vi "Autonomous Independent.vi"() -> ()   [LabVIEW 2023]
doc: "This VI is called when autonomous begins, and will automatically be terminated when autonomous ends. You can carry out timed or sensor driven robot movement independently without needing to return to the caller."
uses:
  ctrl defs/ctrl robot swerve dims.ctl
  ctrl defs/ctrl AUTO SIMPLE STEP.ctl
  <vilib>/Rock Robotics/WPI/Utilities/WPI_GetSetVariantRefNum.vi
  <vilib>/Rock Robotics/Network Tables/NT Read String.vi
  <vilib>/Rock Robotics/Network Tables/NT Write Numeric Array.vi
  Global odometry.vi
  Global INIT.vi
  <vilib>/Rock Robotics/WPI/ThirdParty/JAS_Junk/TrajLib/Trajectory_Library.lvlib
  <vilib>/Rock Robotics/Network Tables/NT Write Boolean.vi
panel:
  in  "Tab Control":T1(tab)
  in  "leg 1 distance (ft)":dbl=1.06 format="%#_13g"
  in  "leg 1\nVBus":dbl=0.5 format="%#_13g"
  in  "leg 2 distance (ft)":dbl=8.0 format="%#_13g"
  in  "leg 2\nVBus":dbl=0.5 format="%#_13g"
  in  "DRIVE BRNG (deg)":dbl=60.0 min=0.0 max=90.0 format="%#_13g"
  in  "DRIVE CTR-STAGE (ft)":dbl=15.0 caption="distance wall to center stage (in feet)" min=0.02 max=27.0 step=0.02 format="%.2f"
  in  "DRIVE CTR-STAGE %VBus":dbl=0.5499999999999999 caption="drive center-stage throttle %" min=0.02 max=0.7 step=0.01 format="%.2f"
  in  "DRIVE MID-CT (ft)":dbl=25.76 caption="distance wall to mid-court (in feet)" min=0.02 max=27.0 step=0.02 format="%.2f"
  in  "DRIVE MID-CT %VBus":dbl=0.65 caption="drive mid-court throttle %" min=0.02 max=0.7 step=0.01 format="%.2f"
  in  "DRIVE OUT %VBus":dbl=0.5 caption="drive away throttle %" min=0.02 max=0.7 step=0.01 format="%.2f"
  in  "DRIVE OUT (ft)":dbl=8.0 caption="SPEAKER front to NOTE (in feet)" min=0.02 max=25.0 step=0.02 format="%.2f"
  in  "delay to wait to\nSHOOT (ms)":u32=1500
  in  "pause after\ndrive out (ms)":u32=500
  in  "DRIVE IN (ft)":dbl=8.0 caption="distance to return to SPEAKER (in feet)" min=0.02 max=25.0 step=0.02 format="%.2f"
  in  "DRIVE IN %VBus":dbl=0.4 caption="drive return throttle %" min=0.02 max=0.7 step=0.01 format="%.2f"
  out "ROBOT frame dims":T2={"width"=30.0, "depth"=30.0}
  in  "bumper thickness (in)":dbl=3.25 format="%#_13g"
  out "POS after (rev)":dbl[](array[numeric])
  out "POS start (rev)":dbl[](array[numeric])
  out "distance\ntravel (in)":dbl[](array[numeric])
  out "revs moved":dbl[](array[numeric])
  out "inches\nper rev":dbl
  out "YRPHfH start":T3={"Yaw"=129.52, "Roll"=0.02, "Pitch"=-0.05, "Heading"=270.74, "Fused Heading"=129.25}
  out "YRPHfH after first leg":T3={"Yaw"=129.52, "Roll"=0.02, "Pitch"=-0.05, "Heading"=270.74, "Fused Heading"=129.25}
  out "YRPHfH end":T3={"Yaw"=129.52, "Roll"=0.02, "Pitch"=-0.05, "Heading"=270.74, "Fused Heading"=129.25}
  out "overall change":T3
  out "change from leg 1 to 2":T3
  out "Milliseconds":u16
  out "av vel (in/s)":dbl[](array[numeric])
  # "ANGLED PROGRAMS from SUB-WOOFER sides"
  # "DISTANCES:\n\nGO-LINE:\n    6.34 ft from driver's wall\n    3.33 ft from sub-woofer\n\nNOTE line:\n    9.67 ft from driver's wall\n    6.65 ft from sub-woofer\n\nCENTER-STAGE line:\n    19.27 ft from driver's wall\n\nMID-COURT:\n     27.22 ft from driver's wall\n\nROBOT is 30 x 30 with 3.5\" bumpers\n37 x 37 overall; 18.5\" to center"
  # "Be sure to right-click and choose Data Operations>>Make Current Value default if you want to save the array values with the VI"
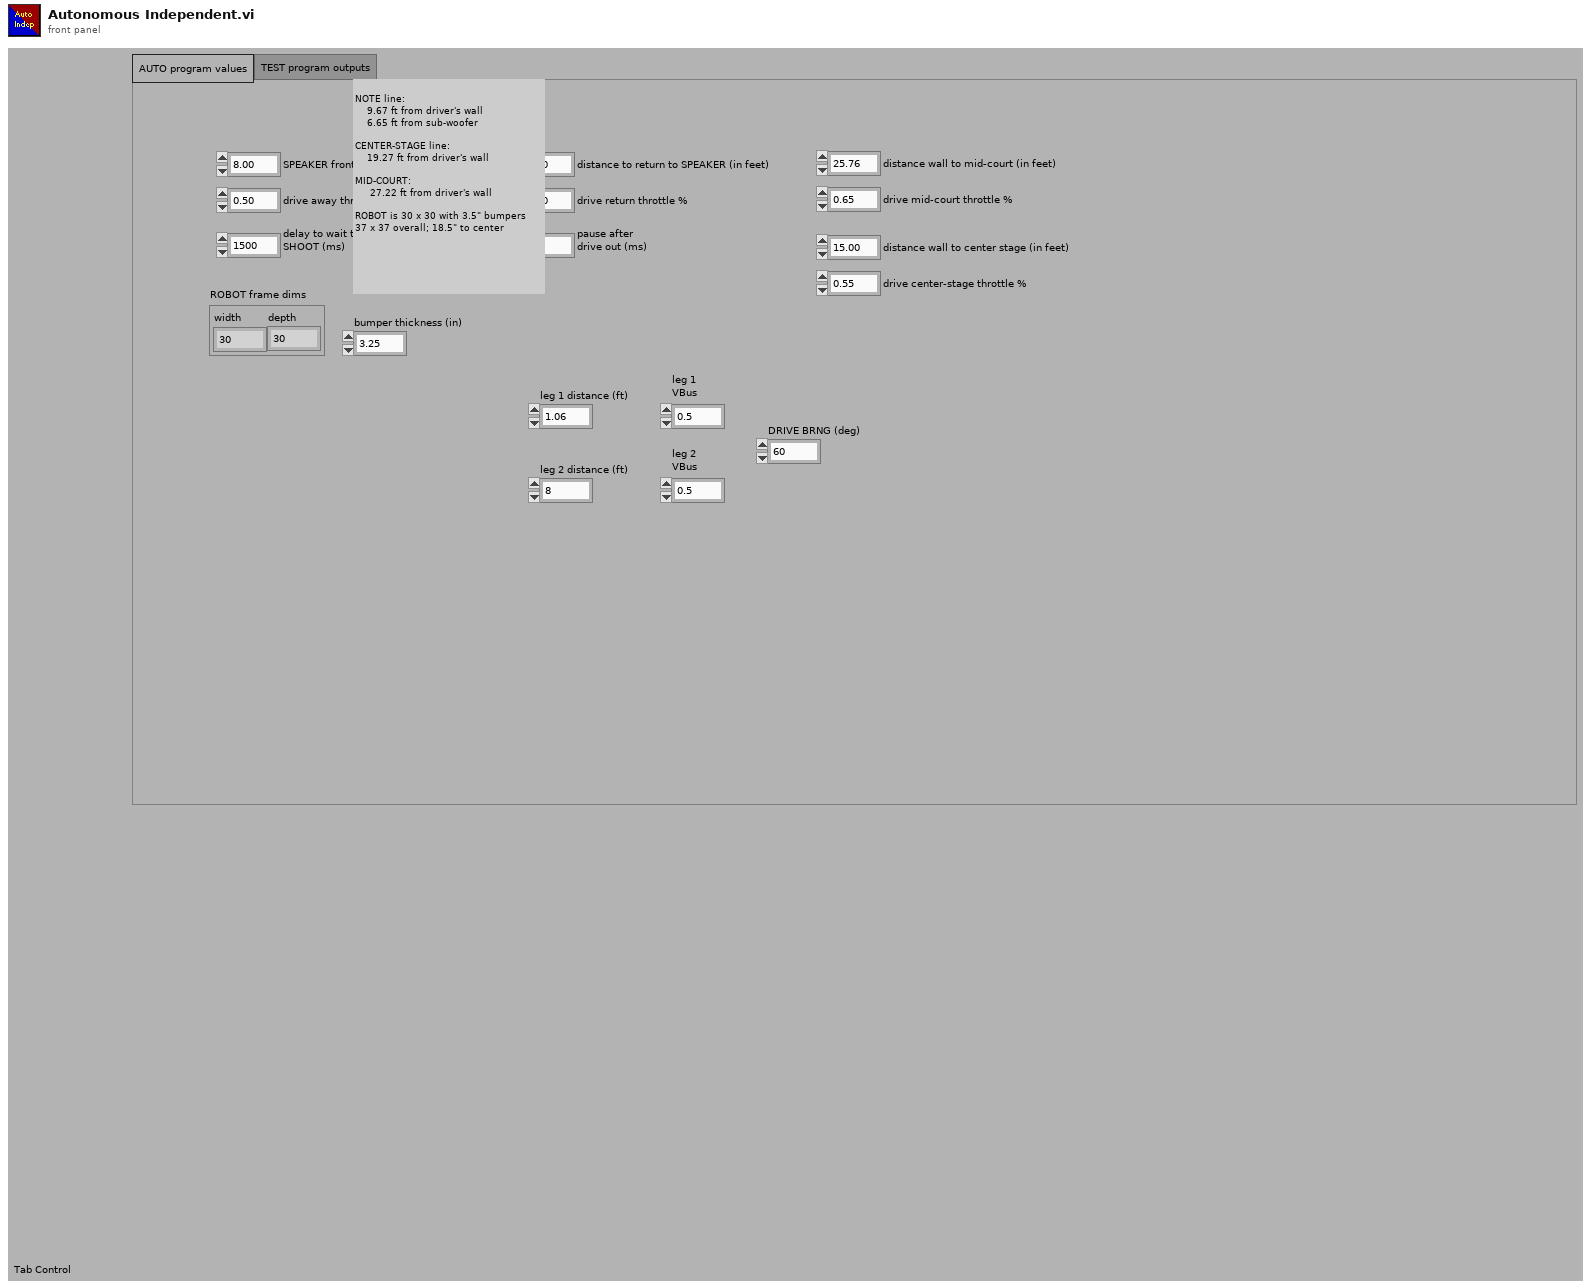
[diagram p1: front panel]
types:
  T1 = enum32{"AUTO program values", "TEST program outputs"}
  T2 = typedef "ctrl robot swerve dims.ctl" = cluster{"width":dbl, "depth":dbl}
  T3 = cluster{"Yaw":dbl, "Roll":dbl, "Pitch":dbl, "Heading":dbl, "Fused Heading":dbl}
  T4 = typedef "WPI_JoystickDevRef.ctl" = cluster{"Device":T5}
  T5 = typedef "WPI_JoystickDeviceEnum.ctl" = enum16{"USB 0", "USB 1", "USB 2", "USB 3", "USB 4", "USB 5"}
  T6 = typedef "ctrl AUTO SIMPLE STEP.ctl" = cluster{"SHOOT\nFIRST":bool, "wait to\nSHOOT (ms)":u32, "run\nINTAKE":bool, "DRIVE BRNG (deg)":dbl, "DRIVE OUT\nVBus":dbl, "TIME to\nDRIVE OUT (ms)":u32, "pause after\ndrive out (ms)":u32, "SHOOT\nAGAIN":bool, "DRIVE IN\nVBus":dbl, "TIME to\nDRIVE IN (ms)":u32}
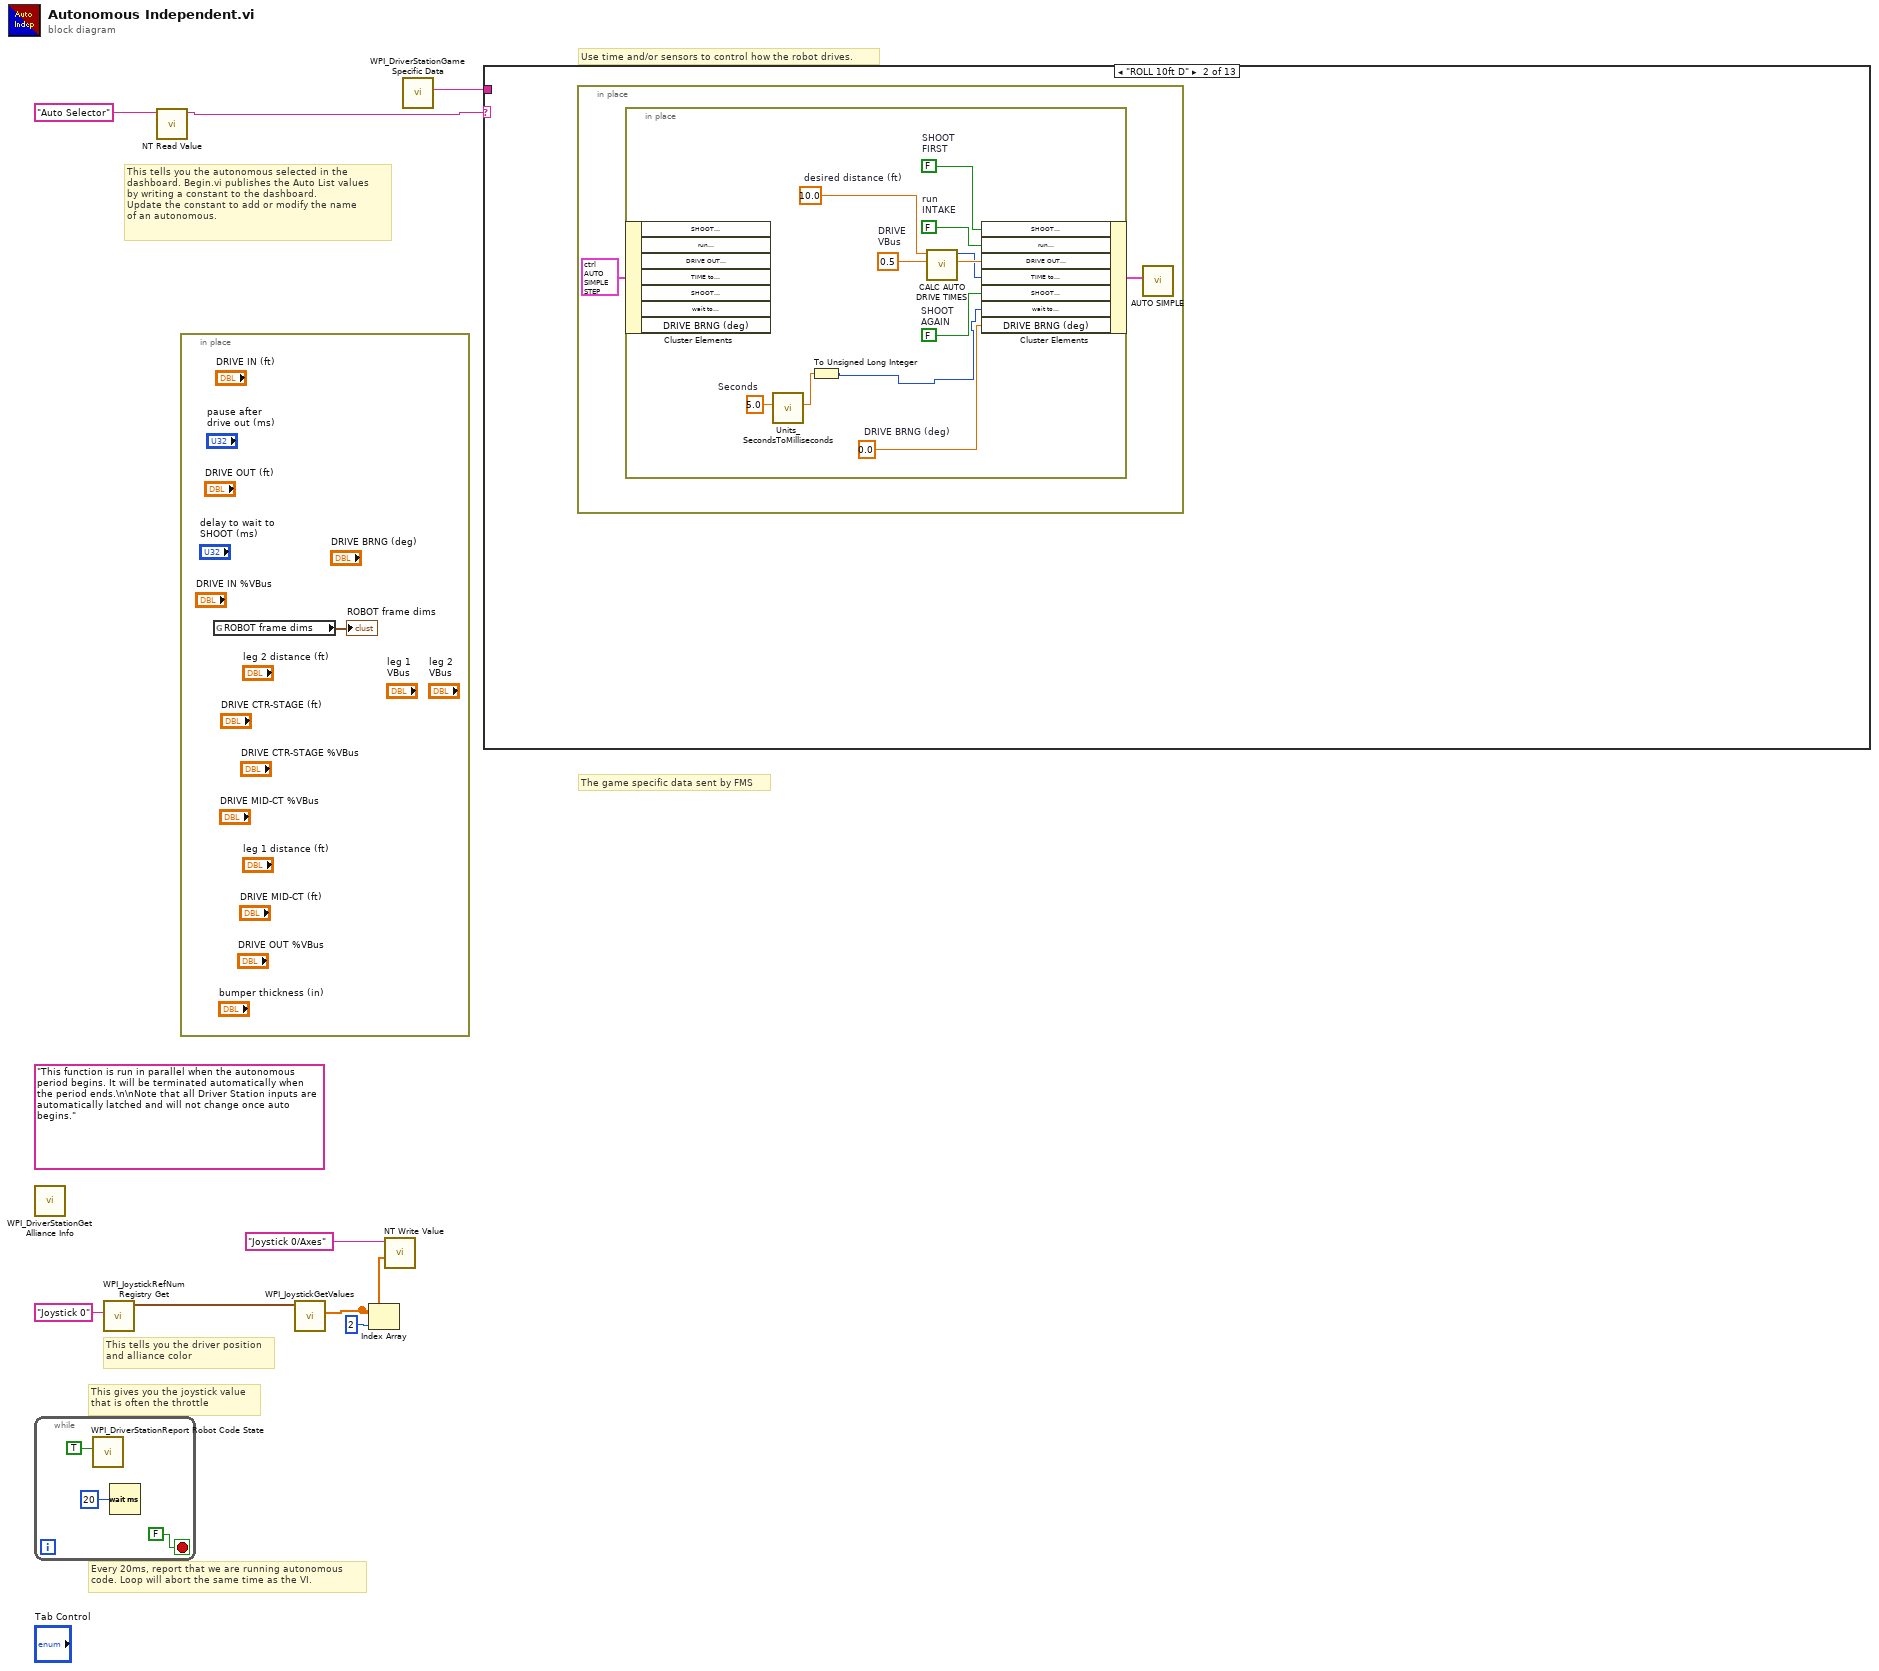
[diagram p0: block diagram]
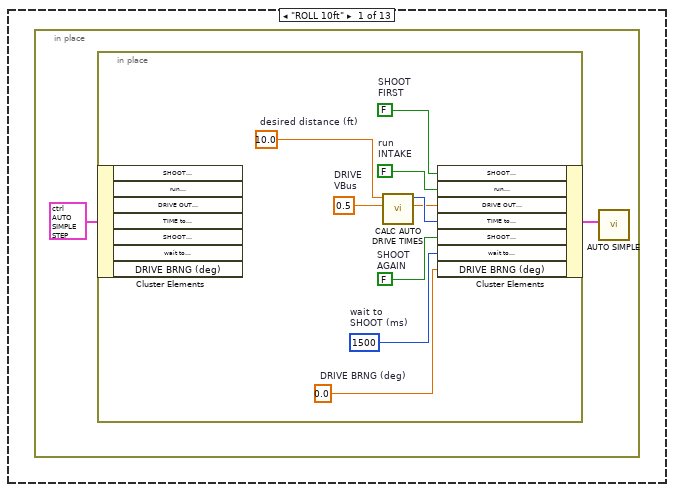
[diagram p2: hidden frame]
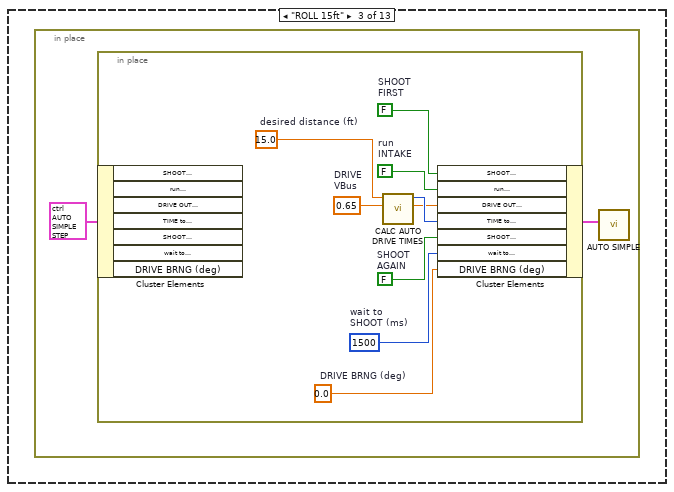
[diagram p3: hidden frame]
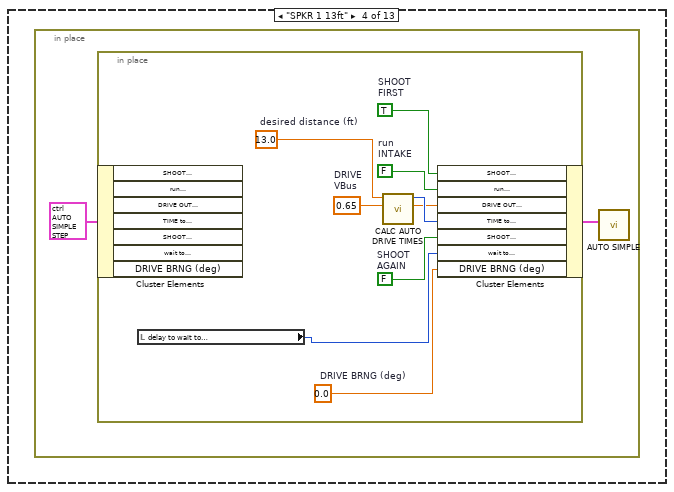
[diagram p4: hidden frame]
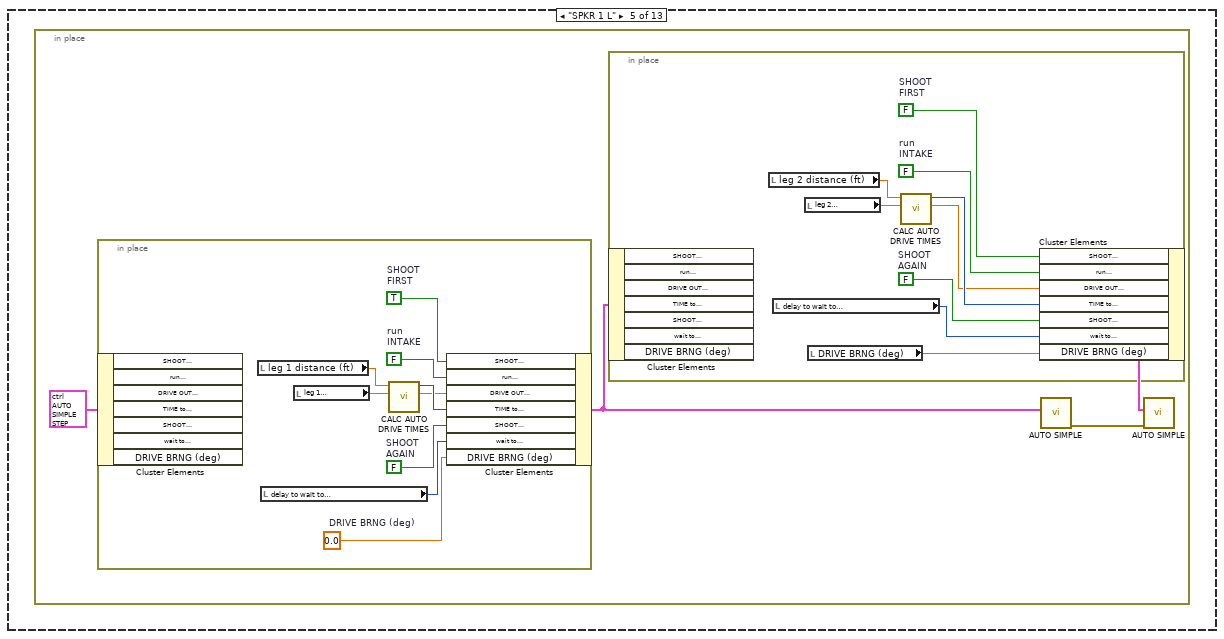
[diagram p5: hidden frame]
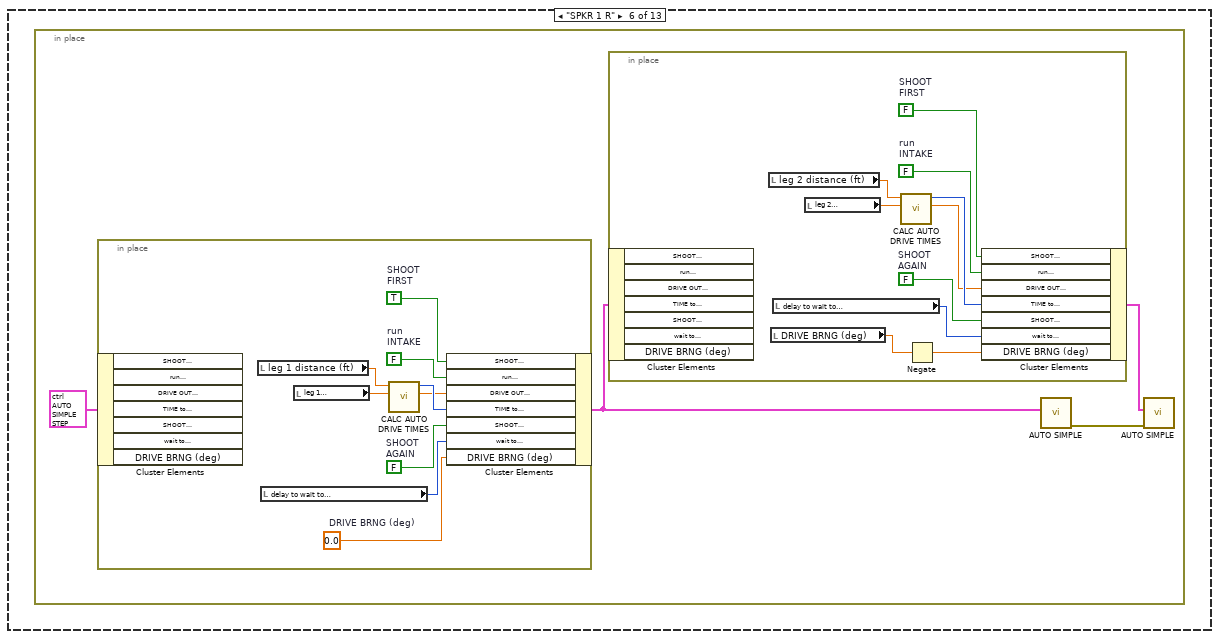
[diagram p6: hidden frame]
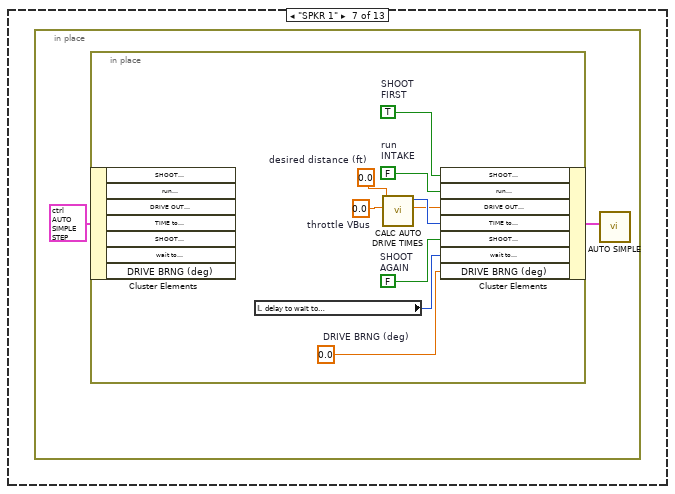
[diagram p7: hidden frame]
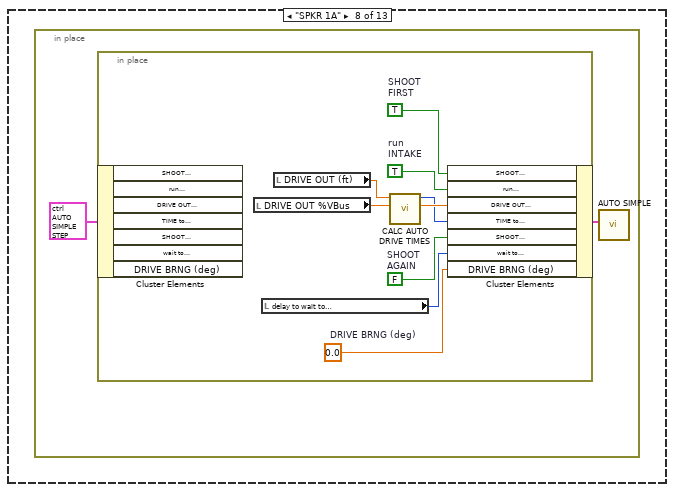
[diagram p8: hidden frame]
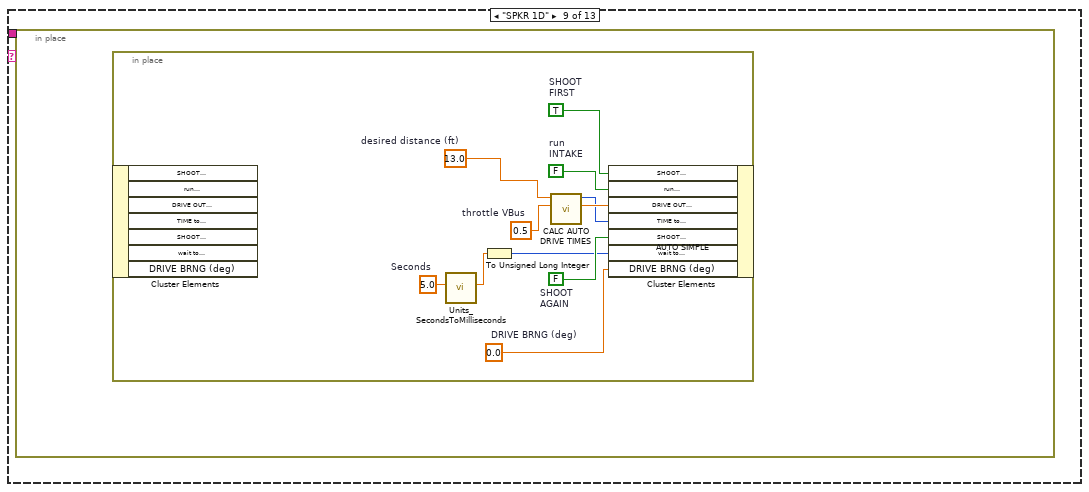
[diagram p9: hidden frame]
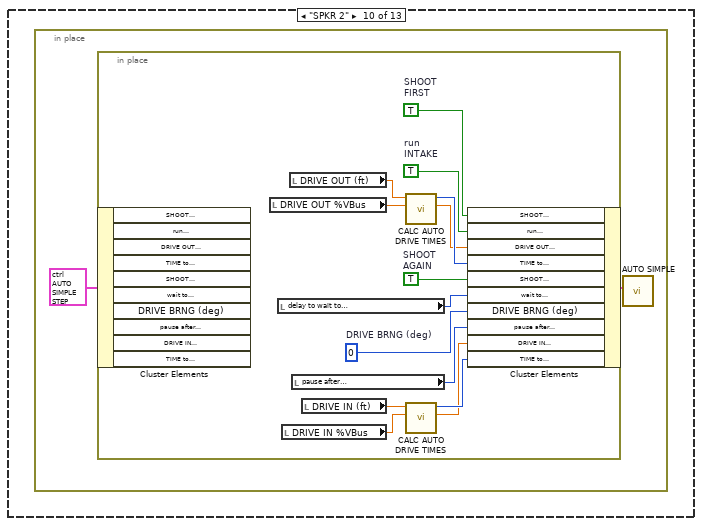
[diagram p10: hidden frame]
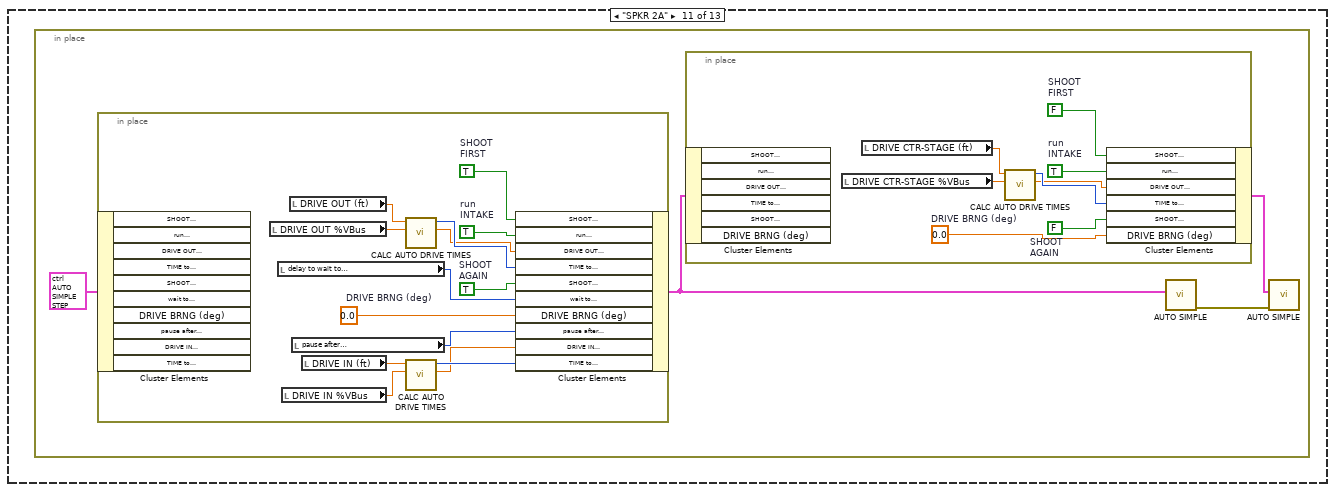
[diagram p11: hidden frame]
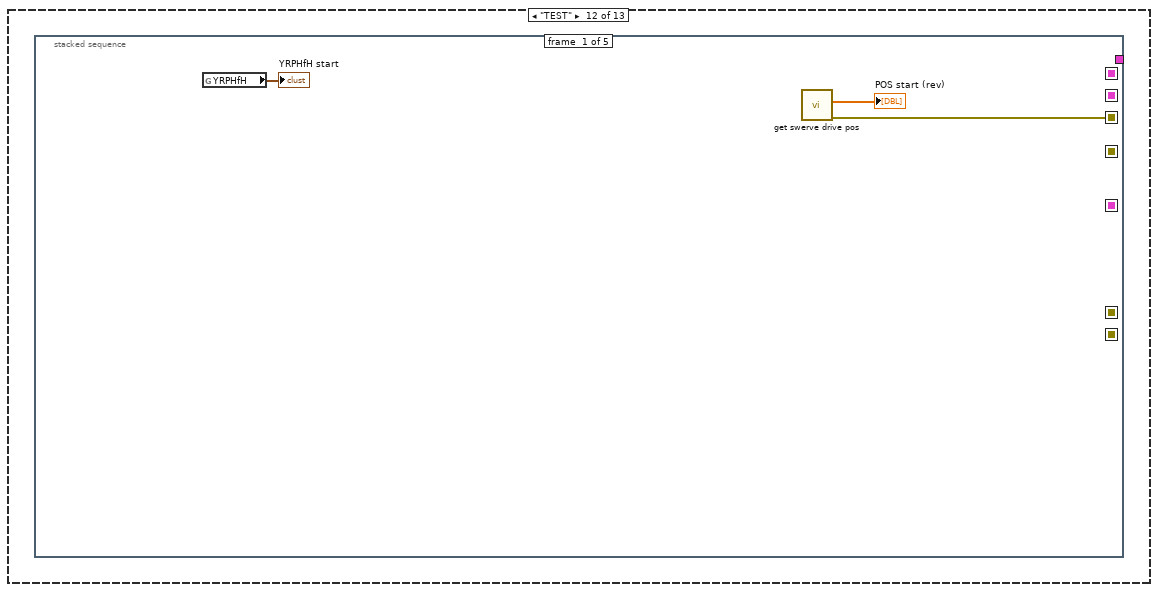
[diagram p12: hidden frame]
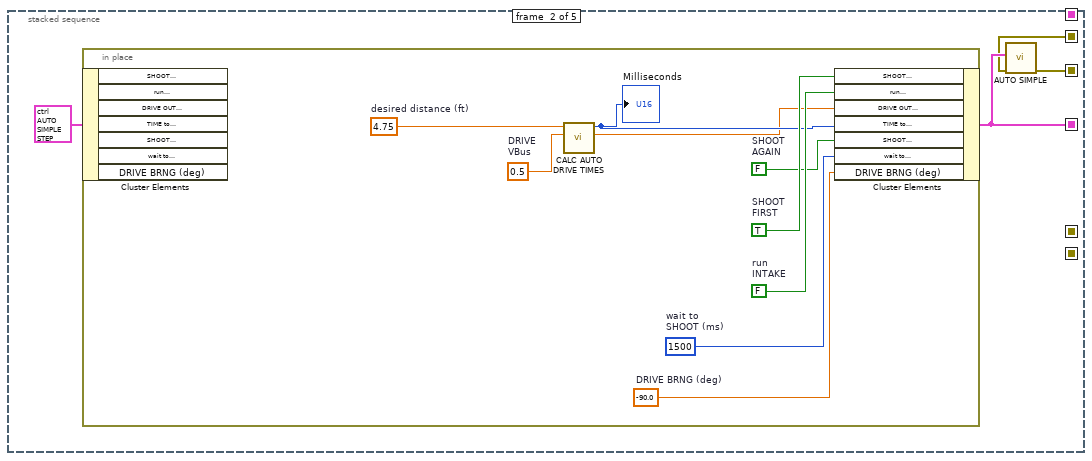
[diagram p13: hidden frame]
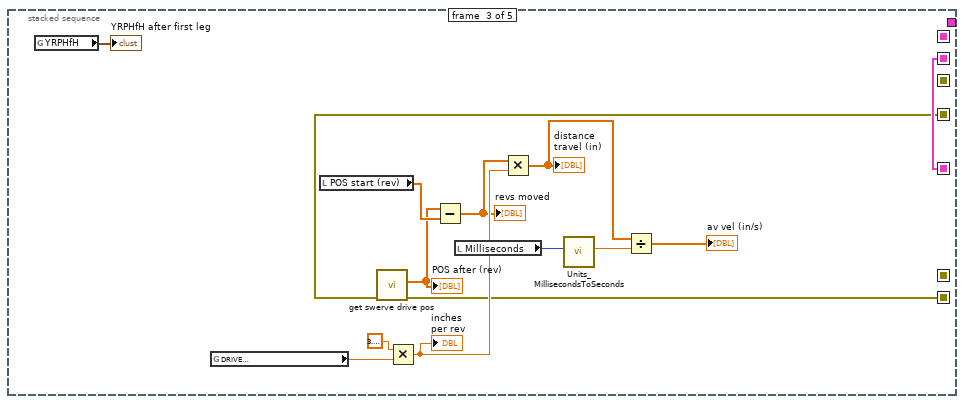
[diagram p14: hidden frame]
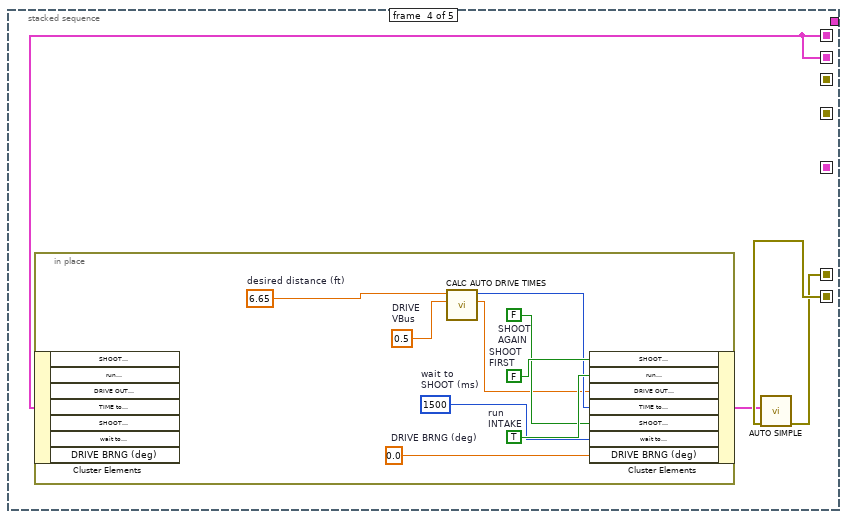
[diagram p15: hidden frame]
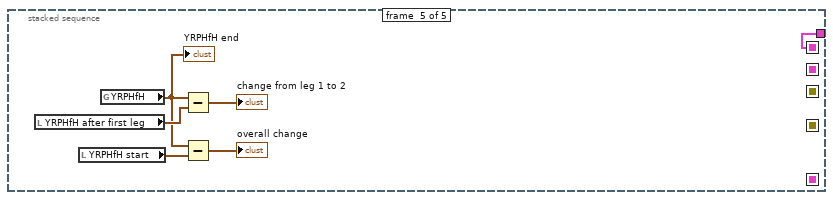
[diagram p16: hidden frame]
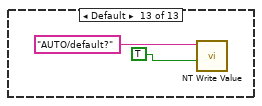
[diagram p17: hidden frame]
diagram:
  (unwired) "This function is run in parallel when the autonomous period begins. It will be terminated automatically when the period ends.\n\nNote that all Driver Station inputs are automatically latched and will not change once auto begins."
  # "The game specific data sent by FMS"
  # "This tells you the autonomous selected in the \ndashboard. Begin.vi publishes the Auto List values\nby writing a constant to the dashboard.\nUpdate the constant to add or modify the name\nof an autonomous."
  # "Every 20ms, report that we are running autonomous\ncode. Loop will abort the same time as the VI."
  # "This gives you the joystick value\nthat is often the throttle"
  # "Use time and/or sensors to control how the robot drives."
  # "This tells you the driver position\nand alliance color"
  n1 = call <vilib>:"WPI_DriverStationGet Alliance Info.vi"() -> ()  [unwired: 12 out]
  n2 = while {
    stop <- FALSE stop-if-true
    n3 = call <vilib>:"WPI_DriverStationReport Robot Code State.vi"("Autonomous"=TRUE) -> ()  [unwired: 10 in, 1 out]
    n4 = Wait (ms)(milliseconds to wait=u32 20) -> ()  [unwired: 1 out]
  }
  n5 = call <vilib>:"WPI_JoystickRefNum Registry Get.vi"("refnum name"="Joystick 0") -> ("JoystickDevRef"=w7:T4)  [unwired: 1 in, 9 out]
  n6 = call-poly <vilib>:"NT Read Value.vi"("name"="Auto Selector" ("Name")) -> ("value"=w4:string)  [unwired: 8 in, 2 out]
  n7 = in-place {
    n8 = global read "Global INIT.vi" "ROBOT frame dims"() -> (→"ROBOT frame dims":T2)
  }
  n9 = call <vilib>:"WPI_JoystickGetValues.vi"("JoystickDevRef"=w7) -> ("Axes"=w3:dbl[])  [unwired: 6 in, 4 out]
  n10 = Index Array(array=w3, index=2) -> ()  [unwired: 1 out]
  n11 = call-poly <vilib>:"NT Write Value.vi"("value"=w3, "name"="Joystick 0/Axes" ("Name")) -> ()  [unwired: 9 in, 1 out]
  n12 = call <vilib>:"WPI_DriverStationGame Specific Data.vi"() -> ("Game Specific Data"=w1:string)  [unwired: 11 in]
  n13 = case shown="\"ROLL 10ft D\"" w4 {
    tunnel: w1 -> [_ _ _ _ _ _ _ _ _ _ _ _ _]
    frame "ROLL 10ft" {
      n14 = in-place {
        n15 = in-place {
          w15 = 0.0  # DRIVE BRNG (deg)
          w17 = 10.0  # desired distance (ft)
          w21 = u32 1500  # wait to SHOOT (ms)
          w18 = 0.5  # DRIVE VBus
          w20 = FALSE  # SHOOT AGAIN
          w22 = FALSE  # run INTAKE
          w23 = FALSE  # SHOOT FIRST
          n16 = in-place-cluster #1(T6 {"SHOOT\nFIRST"=FALSE, "wait to\nSHOOT (ms)"=1500, "run\nINTAKE"=FALSE, "DRIVE BRNG (deg)"=1750.0, "DRIVE OUT\nVBus"=0.65, "TIME to\nDRIVE OUT (ms)"=1750, "pause after\ndrive out (ms)"=1750, "SHOOT\nAGAIN"=FALSE, "DRIVE IN\nVBus"=0.65, "TIME to\nDRIVE IN (ms)"=1750} ("Cluster")) -> ()  [unwired: 7 out]
          n17 = call "CALC AUTO DRIVE TIMES.vi"("throttle VBus"=w18, "desired distance (ft)"=w17) -> ("throttle out"=w16:dbl, "Milliseconds"=w19:u16)  [unwired: 6 in, 2 out]
          n18 = in-place-cluster #1("SHOOT\nFIRST"=w23, "run\nINTAKE"=w22, "DRIVE OUT\nVBus"=w16, "TIME to\nDRIVE OUT (ms)"=w19, "SHOOT\nAGAIN"=w20, "wait to\nSHOOT (ms)"=w21, "DRIVE BRNG (deg)"=w15) -> (w14:T6)
        }
        n19 = call "AUTO SIMPLE.vi"("auto command list"=w14) -> ()  [unwired: 10 in, 1 out]
      }
    }
    frame "ROLL 10ft D" {
      n20 = in-place {
        n21 = in-place {
          w27 = 5.0  # Seconds
          w30 = 0.0  # DRIVE BRNG (deg)
          w32 = 10.0  # desired distance (ft)
          w33 = 0.5  # DRIVE VBus
          w34 = FALSE  # SHOOT AGAIN
          w35 = FALSE  # run INTAKE
          w36 = FALSE  # SHOOT FIRST
          n22 = in-place-cluster #2(T6 {"SHOOT\nFIRST"=FALSE, "wait to\nSHOOT (ms)"=1500, "run\nINTAKE"=FALSE, "DRIVE BRNG (deg)"=1750.0, "DRIVE OUT\nVBus"=0.65, "TIME to\nDRIVE OUT (ms)"=1750, "pause after\ndrive out (ms)"=1750, "SHOOT\nAGAIN"=FALSE, "DRIVE IN\nVBus"=0.65, "TIME to\nDRIVE IN (ms)"=1750} ("Cluster")) -> ()  [unwired: 7 out]
          n23 = call <vilib>:"Units_SecondsToMilliseconds.vi"("Seconds"=w27) -> ("Milliseconds"=w28:dbl)  [unwired: 10 in]
          n24 = To Unsigned Long Integer(number=w28) -> (unsigned 32bit integer=w26:u32)
          n25 = call "CALC AUTO DRIVE TIMES.vi"("throttle VBus"=w33, "desired distance (ft)"=w32) -> ("throttle out"=w31:dbl, "Milliseconds"=w29:u16)  [unwired: 6 in, 2 out]
          n26 = in-place-cluster #2("SHOOT\nFIRST"=w36, "run\nINTAKE"=w35, "DRIVE OUT\nVBus"=w31, "TIME to\nDRIVE OUT (ms)"=w29, "SHOOT\nAGAIN"=w34, "wait to\nSHOOT (ms)"=w26, "DRIVE BRNG (deg)"=w30) -> (w25:T6)
        }
        n27 = call "AUTO SIMPLE.vi"("auto command list"=w25) -> ()  [unwired: 10 in, 1 out]
      }
    }
    frame "ROLL 15ft" {
      n28 = in-place {
        n29 = in-place {
          w39 = 0.0  # DRIVE BRNG (deg)
          w41 = 15.0  # desired distance (ft)
          w45 = u32 1500  # wait to SHOOT (ms)
          w42 = 0.65  # DRIVE VBus
          w44 = FALSE  # SHOOT AGAIN
          w46 = FALSE  # run INTAKE
          w47 = FALSE  # SHOOT FIRST
          n30 = in-place-cluster #3(T6 {"SHOOT\nFIRST"=FALSE, "wait to\nSHOOT (ms)"=1500, "run\nINTAKE"=FALSE, "DRIVE BRNG (deg)"=1750.0, "DRIVE OUT\nVBus"=0.65, "TIME to\nDRIVE OUT (ms)"=1750, "pause after\ndrive out (ms)"=1750, "SHOOT\nAGAIN"=FALSE, "DRIVE IN\nVBus"=0.65, "TIME to\nDRIVE IN (ms)"=1750} ("Cluster")) -> ()  [unwired: 7 out]
          n31 = call "CALC AUTO DRIVE TIMES.vi"("throttle VBus"=w42, "desired distance (ft)"=w41) -> ("throttle out"=w40:dbl, "Milliseconds"=w43:u16)  [unwired: 6 in, 2 out]
          n32 = in-place-cluster #3("SHOOT\nFIRST"=w47, "run\nINTAKE"=w46, "DRIVE OUT\nVBus"=w40, "TIME to\nDRIVE OUT (ms)"=w43, "SHOOT\nAGAIN"=w44, "wait to\nSHOOT (ms)"=w45, "DRIVE BRNG (deg)"=w39) -> (w38:T6)
        }
        n33 = call "AUTO SIMPLE.vi"("auto command list"=w38) -> ()  [unwired: 10 in, 1 out]
      }
    }
    frame "SPKR 1 13ft" {
      n34 = in-place {
        n35 = in-place {
          w51 = 0.0  # DRIVE BRNG (deg)
          w53 = 13.0  # desired distance (ft)
          w54 = 0.65  # DRIVE VBus
          w56 = FALSE  # SHOOT AGAIN
          w57 = FALSE  # run INTAKE
          w58 = TRUE  # SHOOT FIRST
          n36 = in-place-cluster #4(T6 {"SHOOT\nFIRST"=FALSE, "wait to\nSHOOT (ms)"=1500, "run\nINTAKE"=FALSE, "DRIVE BRNG (deg)"=1750.0, "DRIVE OUT\nVBus"=0.65, "TIME to\nDRIVE OUT (ms)"=1750, "pause after\ndrive out (ms)"=1750, "SHOOT\nAGAIN"=FALSE, "DRIVE IN\nVBus"=0.65, "TIME to\nDRIVE IN (ms)"=1750} ("Cluster")) -> ()  [unwired: 7 out]
          n37 = local read "delay to wait to\nSHOOT (ms)"() -> (w50:u32)
          n38 = call "CALC AUTO DRIVE TIMES.vi"("throttle VBus"=w54, "desired distance (ft)"=w53) -> ("throttle out"=w52:dbl, "Milliseconds"=w55:u16)  [unwired: 6 in, 2 out]
          n39 = in-place-cluster #4("SHOOT\nFIRST"=w58, "run\nINTAKE"=w57, "DRIVE OUT\nVBus"=w52, "TIME to\nDRIVE OUT (ms)"=w55, "SHOOT\nAGAIN"=w56, "wait to\nSHOOT (ms)"=w50, "DRIVE BRNG (deg)"=w51) -> (w49:T6)
        }
        n40 = call "AUTO SIMPLE.vi"("auto command list"=w49) -> ()  [unwired: 10 in, 1 out]
      }
    }
    frame "SPKR 1 L" {
      n41 = in-place {
        n42 = in-place {
          w77 = 0.0  # DRIVE BRNG (deg)
          w78 = FALSE  # SHOOT AGAIN
          w79 = FALSE  # run INTAKE
          w80 = TRUE  # SHOOT FIRST
          n43 = in-place-cluster #5(T6 {"SHOOT\nFIRST"=FALSE, "wait to\nSHOOT (ms)"=1500, "run\nINTAKE"=FALSE, "DRIVE BRNG (deg)"=1750.0, "DRIVE OUT\nVBus"=0.65, "TIME to\nDRIVE OUT (ms)"=1750, "pause after\ndrive out (ms)"=1750, "SHOOT\nAGAIN"=FALSE, "DRIVE IN\nVBus"=0.65, "TIME to\nDRIVE IN (ms)"=1750} ("Cluster")) -> ()  [unwired: 7 out]
          n44 = local read "leg 1 distance (ft)"() -> (w73:dbl)
          n45 = local read "delay to wait to\nSHOOT (ms)"() -> (w72:u32)
          n46 = local read "leg 1\nVBus"() -> (w74:dbl)
          n47 = call "CALC AUTO DRIVE TIMES.vi"("throttle VBus"=w74, "desired distance (ft)"=w73) -> ("throttle out"=w75:dbl, "Milliseconds"=w76:u16)  [unwired: 6 in, 2 out]
          n48 = in-place-cluster #5("SHOOT\nFIRST"=w80, "run\nINTAKE"=w79, "DRIVE OUT\nVBus"=w75, "TIME to\nDRIVE OUT (ms)"=w76, "SHOOT\nAGAIN"=w78, "wait to\nSHOOT (ms)"=w72, "DRIVE BRNG (deg)"=w77) -> (w61:T6)
        }
        n49 = in-place {
          w69 = FALSE  # SHOOT AGAIN
          w70 = FALSE  # run INTAKE
          w71 = FALSE  # SHOOT FIRST
          n50 = in-place-cluster #6(w61) -> ()  [unwired: 7 out]
          n51 = local read "leg 2 distance (ft)"() -> (w65:dbl)
          n52 = local read "delay to wait to\nSHOOT (ms)"() -> (w64:u32)
          n53 = local read "leg 2\nVBus"() -> (w66:dbl)
          n54 = local read "DRIVE BRNG (deg)"() -> (w63:dbl)
          n55 = call "CALC AUTO DRIVE TIMES.vi"("throttle VBus"=w66, "desired distance (ft)"=w65) -> ("throttle out"=w67:dbl, "Milliseconds"=w68:u16)  [unwired: 6 in, 2 out]
          n56 = in-place-cluster #6("SHOOT\nFIRST"=w71, "run\nINTAKE"=w70, "DRIVE OUT\nVBus"=w67, "TIME to\nDRIVE OUT (ms)"=w68, "SHOOT\nAGAIN"=w69, "wait to\nSHOOT (ms)"=w64, "DRIVE BRNG (deg)"=w63) -> (w60:T6)
        }
        n57 = call "AUTO SIMPLE.vi"("auto command list"=w61) -> ("error out"=w59:errorcluster)  [unwired: 10 in]
        n58 = call "AUTO SIMPLE.vi"("error in (no error)"=w59, "auto command list"=w60) -> ()  [unwired: 9 in, 1 out]
      }
    }
    frame "SPKR 1 R" {
      n59 = in-place {
        n60 = in-place {
          w100 = 0.0  # DRIVE BRNG (deg)
          w101 = FALSE  # SHOOT AGAIN
          w102 = FALSE  # run INTAKE
          w103 = TRUE  # SHOOT FIRST
          n61 = in-place-cluster #7(T6 {"SHOOT\nFIRST"=FALSE, "wait to\nSHOOT (ms)"=1500, "run\nINTAKE"=FALSE, "DRIVE BRNG (deg)"=1750.0, "DRIVE OUT\nVBus"=0.65, "TIME to\nDRIVE OUT (ms)"=1750, "pause after\ndrive out (ms)"=1750, "SHOOT\nAGAIN"=FALSE, "DRIVE IN\nVBus"=0.65, "TIME to\nDRIVE IN (ms)"=1750} ("Cluster")) -> ()  [unwired: 7 out]
          n62 = local read "leg 1 distance (ft)"() -> (w95:dbl)
          n63 = local read "delay to wait to\nSHOOT (ms)"() -> (w97:u32)
          n64 = local read "leg 1\nVBus"() -> (w96:dbl)
          n65 = call "CALC AUTO DRIVE TIMES.vi"("throttle VBus"=w96, "desired distance (ft)"=w95) -> ("throttle out"=w98:dbl, "Milliseconds"=w99:u16)  [unwired: 6 in, 2 out]
          n66 = in-place-cluster #7("SHOOT\nFIRST"=w103, "run\nINTAKE"=w102, "DRIVE OUT\nVBus"=w98, "TIME to\nDRIVE OUT (ms)"=w99, "SHOOT\nAGAIN"=w101, "wait to\nSHOOT (ms)"=w97, "DRIVE BRNG (deg)"=w100) -> (w83:T6)
        }
        n67 = in-place {
          w92 = FALSE  # SHOOT AGAIN
          w93 = FALSE  # run INTAKE
          w94 = FALSE  # SHOOT FIRST
          n68 = in-place-cluster #8(w83) -> ()  [unwired: 7 out]
          n69 = local read "leg 2 distance (ft)"() -> (w87:dbl)
          n70 = local read "DRIVE BRNG (deg)"() -> (w86:dbl)
          n71 = local read "delay to wait to\nSHOOT (ms)"() -> (w89:u32)
          n72 = local read "leg 2\nVBus"() -> (w88:dbl)
          n73 = call "CALC AUTO DRIVE TIMES.vi"("throttle VBus"=w88, "desired distance (ft)"=w87) -> ("throttle out"=w90:dbl, "Milliseconds"=w91:u16)  [unwired: 6 in, 2 out]
          n74 = Negate(x=w86) -> (-x=w85:dbl)
          n75 = in-place-cluster #8("SHOOT\nFIRST"=w94, "run\nINTAKE"=w93, "DRIVE OUT\nVBus"=w90, "TIME to\nDRIVE OUT (ms)"=w91, "SHOOT\nAGAIN"=w92, "wait to\nSHOOT (ms)"=w89, "DRIVE BRNG (deg)"=w85) -> (w82:T6)
        }
        n76 = call "AUTO SIMPLE.vi"("auto command list"=w83) -> ("error out"=w81:errorcluster)  [unwired: 10 in]
        n77 = call "AUTO SIMPLE.vi"("error in (no error)"=w81, "auto command list"=w82) -> ()  [unwired: 9 in, 1 out]
      }
    }
    frame "SPKR 1" {
      n78 = in-place {
        n79 = in-place {
          w106 = 0.0  # desired distance (ft)
          w107 = 0.0  # throttle VBus
          w111 = 0.0  # DRIVE BRNG (deg)
          w112 = FALSE  # SHOOT AGAIN
          w113 = FALSE  # run INTAKE
          w114 = TRUE  # SHOOT FIRST
          n80 = in-place-cluster #9(T6 {"SHOOT\nFIRST"=FALSE, "wait to\nSHOOT (ms)"=1500, "run\nINTAKE"=FALSE, "DRIVE BRNG (deg)"=1750.0, "DRIVE OUT\nVBus"=0.65, "TIME to\nDRIVE OUT (ms)"=1750, "pause after\ndrive out (ms)"=1750, "SHOOT\nAGAIN"=FALSE, "DRIVE IN\nVBus"=0.65, "TIME to\nDRIVE IN (ms)"=1750} ("Cluster")) -> ()  [unwired: 7 out]
          n81 = local read "delay to wait to\nSHOOT (ms)"() -> (w108:u32)
          n82 = call "CALC AUTO DRIVE TIMES.vi"("throttle VBus"=w107, "desired distance (ft)"=w106) -> ("throttle out"=w109:dbl, "Milliseconds"=w110:u16)  [unwired: 6 in, 2 out]
          n83 = in-place-cluster #9("SHOOT\nFIRST"=w114, "run\nINTAKE"=w113, "DRIVE OUT\nVBus"=w109, "TIME to\nDRIVE OUT (ms)"=w110, "SHOOT\nAGAIN"=w112, "wait to\nSHOOT (ms)"=w108, "DRIVE BRNG (deg)"=w111) -> (w104:T6)
        }
        n84 = call "AUTO SIMPLE.vi"("auto command list"=w104) -> ()  [unwired: 10 in, 1 out]
      }
    }
    frame "SPKR 1A" {
      n85 = in-place {
        n86 = in-place {
          w120 = 0.0  # DRIVE BRNG (deg)
          w123 = FALSE  # SHOOT AGAIN
          w125 = TRUE  # run INTAKE
          w124 = TRUE  # SHOOT FIRST
          n87 = in-place-cluster #10(T6 {"SHOOT\nFIRST"=FALSE, "wait to\nSHOOT (ms)"=1500, "run\nINTAKE"=FALSE, "DRIVE BRNG (deg)"=1750.0, "DRIVE OUT\nVBus"=0.65, "TIME to\nDRIVE OUT (ms)"=1750, "pause after\ndrive out (ms)"=1750, "SHOOT\nAGAIN"=FALSE, "DRIVE IN\nVBus"=0.65, "TIME to\nDRIVE IN (ms)"=1750} ("Cluster")) -> ()  [unwired: 7 out]
          n88 = local read "DRIVE OUT %VBus"() -> (w118:dbl)
          n89 = local read "delay to wait to\nSHOOT (ms)"() -> (w117:u32)
          n90 = local read "DRIVE OUT (ft)"() -> (w119:dbl)
          n91 = call "CALC AUTO DRIVE TIMES.vi"("throttle VBus"=w118, "desired distance (ft)"=w119) -> ("throttle out"=w122:dbl, "Milliseconds"=w121:u16)  [unwired: 6 in, 2 out]
          n92 = in-place-cluster #10("SHOOT\nFIRST"=w124, "run\nINTAKE"=w125, "DRIVE OUT\nVBus"=w122, "TIME to\nDRIVE OUT (ms)"=w121, "SHOOT\nAGAIN"=w123, "wait to\nSHOOT (ms)"=w117, "DRIVE BRNG (deg)"=w120) -> (w115:T6)
        }
        n93 = call "AUTO SIMPLE.vi"("auto command list"=w115) -> ()  [unwired: 10 in, 1 out]
      }
    }
    frame "SPKR 1D" {
      n94 = in-place {
        n95 = in-place {
          w128 = 0.5  # throttle VBus
          w129 = 13.0  # desired distance (ft)
          w130 = 5.0  # Seconds
          w133 = 0.0  # DRIVE BRNG (deg)
          w136 = FALSE  # SHOOT AGAIN
          w138 = FALSE  # run INTAKE
          w137 = TRUE  # SHOOT FIRST
          n96 = in-place-cluster #11(T6 {"SHOOT\nFIRST"=FALSE, "wait to\nSHOOT (ms)"=1500, "run\nINTAKE"=FALSE, "DRIVE BRNG (deg)"=1750.0, "DRIVE OUT\nVBus"=0.65, "TIME to\nDRIVE OUT (ms)"=1750, "pause after\ndrive out (ms)"=1750, "SHOOT\nAGAIN"=FALSE, "DRIVE IN\nVBus"=0.65, "TIME to\nDRIVE IN (ms)"=1750} ("Cluster")) -> ()  [unwired: 7 out]
          n97 = call <vilib>:"Units_SecondsToMilliseconds.vi"("Seconds"=w130) -> ("Milliseconds"=w132:dbl)  [unwired: 10 in]
          n98 = To Unsigned Long Integer(number=w132) -> (unsigned 32bit integer=w131:u32)
          n99 = call "CALC AUTO DRIVE TIMES.vi"("throttle VBus"=w128, "desired distance (ft)"=w129) -> ("throttle out"=w135:dbl, "Milliseconds"=w134:u16)  [unwired: 6 in, 2 out]
          n100 = in-place-cluster #11("SHOOT\nFIRST"=w137, "run\nINTAKE"=w138, "DRIVE OUT\nVBus"=w135, "TIME to\nDRIVE OUT (ms)"=w134, "SHOOT\nAGAIN"=w136, "wait to\nSHOOT (ms)"=w131, "DRIVE BRNG (deg)"=w133) -> (w126:T6)
        }
        n101 = call "AUTO SIMPLE.vi"("auto command list"=w126) -> ()  [unwired: 10 in, 1 out]
      }
    }
    frame "SPKR 2" {
      n102 = in-place {
        n103 = in-place {
          w149 = u32 0  # DRIVE BRNG (deg)
          w152 = TRUE  # SHOOT AGAIN
          w153 = TRUE  # run INTAKE
          w154 = TRUE  # SHOOT FIRST
          n104 = in-place-cluster #12(T6 {"SHOOT\nFIRST"=FALSE, "wait to\nSHOOT (ms)"=1500, "run\nINTAKE"=FALSE, "DRIVE BRNG (deg)"=1750.0, "DRIVE OUT\nVBus"=0.65, "TIME to\nDRIVE OUT (ms)"=1750, "pause after\ndrive out (ms)"=1750, "SHOOT\nAGAIN"=FALSE, "DRIVE IN\nVBus"=0.65, "TIME to\nDRIVE IN (ms)"=1750} ("Cluster")) -> ()  [unwired: 10 out]
          n105 = local read "DRIVE OUT %VBus"() -> (w145:dbl)
          n106 = local read "delay to wait to\nSHOOT (ms)"() -> (w144:u32)
          n107 = local read "DRIVE IN %VBus"() -> (w142:dbl)
          n108 = local read "DRIVE OUT (ft)"() -> (w146:dbl)
          n109 = local read "pause after\ndrive out (ms)"() -> (w143:u32)
          n110 = local read "DRIVE IN (ft)"() -> (w141:dbl)
          n111 = call "CALC AUTO DRIVE TIMES.vi"("throttle VBus"=w145, "desired distance (ft)"=w146) -> ("throttle out"=w150:dbl, "Milliseconds"=w151:u16)  [unwired: 6 in, 2 out]
          n112 = call "CALC AUTO DRIVE TIMES.vi"("throttle VBus"=w142, "desired distance (ft)"=w141) -> ("throttle out"=w147:dbl, "Milliseconds"=w148:u16)  [unwired: 6 in, 2 out]
          n113 = in-place-cluster #12("SHOOT\nFIRST"=w154, "run\nINTAKE"=w153, "DRIVE OUT\nVBus"=w150, "TIME to\nDRIVE OUT (ms)"=w151, "SHOOT\nAGAIN"=w152, "wait to\nSHOOT (ms)"=w144, "DRIVE BRNG (deg)"=w149, "pause after\ndrive out (ms)"=w143, "DRIVE IN\nVBus"=w147, "TIME to\nDRIVE IN (ms)"=w148) -> (w139:T6)
        }
        n114 = call "AUTO SIMPLE.vi"("auto command list"=w139) -> ()  [unwired: 10 in, 1 out]
      }
    }
    frame "SPKR 2A" {
      n115 = in-place {
        n116 = in-place {
          w175 = 0.0  # DRIVE BRNG (deg)
          w178 = TRUE  # SHOOT AGAIN
          w179 = TRUE  # run INTAKE
          w180 = TRUE  # SHOOT FIRST
          n117 = in-place-cluster #13(T6 {"SHOOT\nFIRST"=FALSE, "wait to\nSHOOT (ms)"=1500, "run\nINTAKE"=FALSE, "DRIVE BRNG (deg)"=1750.0, "DRIVE OUT\nVBus"=0.65, "TIME to\nDRIVE OUT (ms)"=1750, "pause after\ndrive out (ms)"=1750, "SHOOT\nAGAIN"=FALSE, "DRIVE IN\nVBus"=0.65, "TIME to\nDRIVE IN (ms)"=1750} ("Cluster")) -> ()  [unwired: 10 out]
          n118 = local read "DRIVE OUT %VBus"() -> (w168:dbl)
          n119 = local read "delay to wait to\nSHOOT (ms)"() -> (w169:u32)
          n120 = local read "DRIVE IN %VBus"() -> (w172:dbl)
          n121 = local read "DRIVE OUT (ft)"() -> (w167:dbl)
          n122 = local read "pause after\ndrive out (ms)"() -> (w170:u32)
          n123 = local read "DRIVE IN (ft)"() -> (w171:dbl)
          n124 = call "CALC AUTO DRIVE TIMES.vi"("throttle VBus"=w168, "desired distance (ft)"=w167) -> ("throttle out"=w176:dbl, "Milliseconds"=w177:u16)  [unwired: 6 in, 2 out]
          n125 = call "CALC AUTO DRIVE TIMES.vi"("throttle VBus"=w172, "desired distance (ft)"=w171) -> ("throttle out"=w173:dbl, "Milliseconds"=w174:u16)  [unwired: 6 in, 2 out]
          n126 = in-place-cluster #13("SHOOT\nFIRST"=w180, "run\nINTAKE"=w179, "DRIVE OUT\nVBus"=w176, "TIME to\nDRIVE OUT (ms)"=w177, "SHOOT\nAGAIN"=w178, "wait to\nSHOOT (ms)"=w169, "DRIVE BRNG (deg)"=w175, "pause after\ndrive out (ms)"=w170, "DRIVE IN\nVBus"=w173, "TIME to\nDRIVE IN (ms)"=w174) -> (w156:T6)
        }
        n127 = in-place {
          w161 = 0.0  # DRIVE BRNG (deg)
          w164 = FALSE  # SHOOT AGAIN
          w165 = TRUE  # run INTAKE
          w166 = FALSE  # SHOOT FIRST
          n128 = in-place-cluster #14(w156) -> ()  [unwired: 6 out]
          n129 = local read "DRIVE CTR-STAGE %VBus"() -> (w160:dbl)
          n130 = local read "DRIVE CTR-STAGE (ft)"() -> (w159:dbl)
          n131 = call "CALC AUTO DRIVE TIMES.vi"("throttle VBus"=w160, "desired distance (ft)"=w159) -> ("throttle out"=w162:dbl, "Milliseconds"=w163:u16)  [unwired: 6 in, 2 out]
          n132 = in-place-cluster #14("SHOOT\nFIRST"=w166, "run\nINTAKE"=w165, "DRIVE OUT\nVBus"=w162, "TIME to\nDRIVE OUT (ms)"=w163, "SHOOT\nAGAIN"=w164, "DRIVE BRNG (deg)"=w161) -> (w157:T6)
        }
        n133 = call "AUTO SIMPLE.vi"("auto command list"=w156) -> ("error out"=w155:errorcluster)  [unwired: 10 in]
        n134 = call "AUTO SIMPLE.vi"("error in (no error)"=w155, "auto command list"=w157) -> ()  [unwired: 9 in, 1 out]
      }
    }
    frame "TEST" {
      n135 = stacked-sequence {
        seq-local: [w182 _ _ _ _] -> [_ w184 _ _ _]
        seq-local: [_ w186 _ _ _] -> [_ _ w205 _ _]
        seq-local: [_ w185 _ _ _] -> [_ _ w210 _ _]
        seq-local: [_ _ w202 _ _] -> [_ _ _ w213 _]
        seq-local: [_ _ w210 _ _] -> [_ _ _ w214 _]
        seq-local: [_ _ _ w214 _] -> [_ _ _ _ w229]
        seq-local: [_ _ _ w211 _] -> [_ _ _ _ _]
        tunnel: [_ _ _ _ w229] -> _
        frame #0 {
          n136 = global read "Global odometry.vi" "YRPHfH"() -> (→"YRPHfH start":T3)
          n137 = call "get swerve drive pos.vi"() -> ("error out"=w182:errorcluster, "Get POS"=→"POS start (rev)":dbl[])  [unwired: 10 in]
        }
        frame #1 {
          n138 = in-place {
            w190 = 4.75  # desired distance (ft)
            w191 = 0.5  # DRIVE VBus
            w192 = -90.0  # DRIVE BRNG (deg)
            w193 = u32 1500  # wait to SHOOT (ms)
            w194 = FALSE  # SHOOT AGAIN
            w195 = FALSE  # run INTAKE
            w196 = TRUE  # SHOOT FIRST
            n139 = in-place-cluster #15(T6 {"SHOOT\nFIRST"=FALSE, "wait to\nSHOOT (ms)"=1500, "run\nINTAKE"=FALSE, "DRIVE BRNG (deg)"=1750.0, "DRIVE OUT\nVBus"=0.65, "TIME to\nDRIVE OUT (ms)"=1750, "pause after\ndrive out (ms)"=1750, "SHOOT\nAGAIN"=FALSE, "DRIVE IN\nVBus"=0.65, "TIME to\nDRIVE IN (ms)"=1750} ("Cluster")) -> ()  [unwired: 7 out]
            n140 = call "CALC AUTO DRIVE TIMES.vi"("throttle VBus"=w191, "desired distance (ft)"=w190) -> ("throttle out"=w188:dbl, "Milliseconds"=w189:u16)  [unwired: 6 in, 2 out]
            "Milliseconds" <- w189
            n141 = in-place-cluster #15("SHOOT\nFIRST"=w196, "run\nINTAKE"=w195, "DRIVE OUT\nVBus"=w188, "TIME to\nDRIVE OUT (ms)"=w189, "SHOOT\nAGAIN"=w194, "wait to\nSHOOT (ms)"=w193, "DRIVE BRNG (deg)"=w192) -> (w185:T6)
          }
          n142 = call "AUTO SIMPLE.vi"("error in (no error)"=w184, "auto command list"=w185) -> ("error out"=w186:errorcluster)  [unwired: 9 in]
        }
        frame #2 {
          n143 = global read "Global odometry.vi" "YRPHfH"() -> (→"YRPHfH after first leg":T3)
          n144 = global read "Global INIT.vi" "DRIVE\nwheel diam (in)"() -> (w207:dbl)
          n145 = local read "POS start (rev)"() -> (w204:dbl[])
          n146 = call "get swerve drive pos.vi"("error in (no error)"=w205) -> ("error out"=w202:errorcluster, "Get POS"=w203:dbl[])  [unwired: 9 in]
          "POS after (rev)" <- w203
          n147 = Multiply(x=3.141592653589793, y=w207) -> (x*y=w209:dbl)
          "inches\nper rev" <- w209
          n148 = Subtract(x=w203, y=w204) -> (x-y=w208:dbl[])
          "revs moved" <- w208
          n149 = local read "Milliseconds"() -> (w199:u16)
          n150 = Multiply(x=w208, y=w209) -> (x*y=w200:dbl[])
          "distance\ntravel (in)" <- w200
          n151 = call <vilib>:"Units_MillisecondsToSeconds.vi"("Milliseconds"=w199) -> ("Seconds"=w198:dbl)  [unwired: 10 in]
          n152 = Divide(x=w200, y=w198) -> (x/y=→"av vel (in/s)":dbl[])
        }
        frame #3 {
          n153 = in-place {
            w217 = 6.65  # desired distance (ft)
            w218 = 0.5  # DRIVE VBus
            w219 = 0.0  # DRIVE BRNG (deg)
            w220 = u32 1500  # wait to SHOOT (ms)
            w221 = FALSE  # SHOOT AGAIN
            w222 = TRUE  # run INTAKE
            w223 = FALSE  # SHOOT FIRST
            n154 = in-place-cluster #16(w214) -> ()  [unwired: 7 out]
            n155 = call "CALC AUTO DRIVE TIMES.vi"("throttle VBus"=w218, "desired distance (ft)"=w217) -> ("throttle out"=w215:dbl, "Milliseconds"=w216:u16)  [unwired: 6 in, 2 out]
            n156 = in-place-cluster #16("SHOOT\nFIRST"=w223, "run\nINTAKE"=w222, "DRIVE OUT\nVBus"=w215, "TIME to\nDRIVE OUT (ms)"=w216, "SHOOT\nAGAIN"=w221, "wait to\nSHOOT (ms)"=w220, "DRIVE BRNG (deg)"=w219) -> (w212:T6)
          }
          n157 = call "AUTO SIMPLE.vi"("error in (no error)"=w213, "auto command list"=w212) -> ("error out"=w211:errorcluster)  [unwired: 9 in]
        }
        frame #4 {
          n158 = local read "YRPHfH after first leg"() -> (w228:T3)
          n159 = local read "YRPHfH start"() -> (w226:T3)
          n160 = global read "Global odometry.vi" "YRPHfH"() -> (w227:T3)
          "YRPHfH end" <- w227
          n161 = Subtract(x=w227, y=w228) -> (x-y=→"change from leg 1 to 2":T3)
          n162 = Subtract(x=w227, y=w226) -> (x-y=→"overall change":T3)
        }
      }
    }
    frame Default {
      n163 = call-poly <vilib>:"NT Write Value.vi"("value"=TRUE, "name"="AUTO/default?") -> ()  [unwired: 9 in, 1 out]
    }
  }
